vi "hardware_close_hardware.vi"(8 "error in (no error)":errorcluster, 11 "newport_xps in":refnum<class "newport_xps.lvclass">) -> (0 "error out":errorcluster, 3 "newport_xps out":refnum<class "newport_xps.lvclass">)   [LabVIEW 2015, in "newport_xps.lvclass"]
uses:
  newport_xps.lvclass
  newport_xps.lvclass/newport_xps.ctl
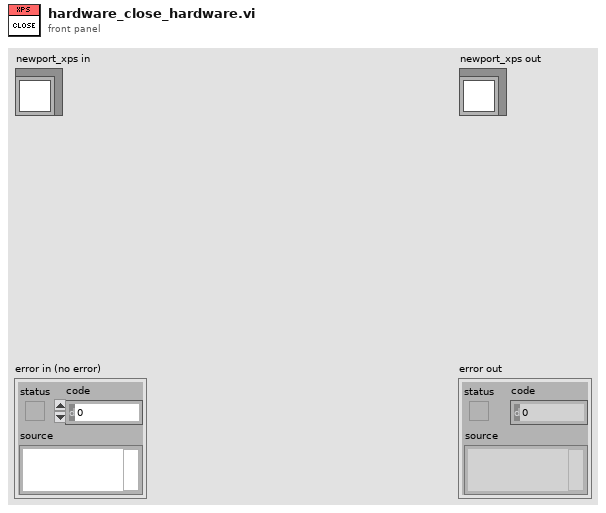
[diagram p1: front panel]
types:
  T1 = cluster{"connection TCP":refnum<k5>, "LogTo File":bool, "Log File refnum":refnum<file>, "no error if error log":bool}
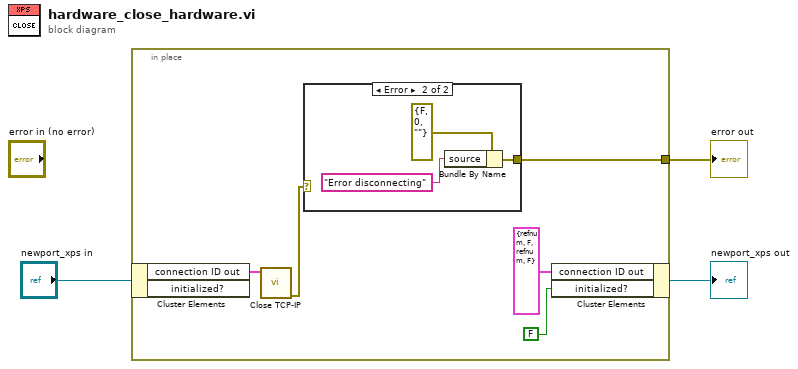
[diagram p0: block diagram]
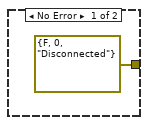
[diagram p2: hidden frame]
diagram:
  n1 = in-place {
    in-place-border: [w4] -> w2
    n2 = in-place-cluster #1("newport_xps in") -> ("connection ID out"=w8:T1)  [unwired: 1 out]
    n3 = call "Close TCP-IP.vi"("connection ID in"=w8) -> ("Error out"=w5:errorcluster)  [unwired: 10 in]
    n4 = case shown="Error" w5 {
      tunnel: [errorcluster {"status"=FALSE, "code"=0, "source"="Disconnected"} ("error IO") w11] -> w4
      frame No Error {
      }
      frame Error {
        n5 = Bundle By Name(cluster=errorcluster {"status"=FALSE, "code"=0, "source"=""} ("error IO"), "source"="Error disconnecting") -> (w11:errorcluster)
      }
    }
    n6 = in-place-cluster #1("connection ID out"=T1 {"connection TCP"=refnum, "LogTo File"=FALSE, "Log File refnum"=refnum, "no error if error log"=FALSE}, "initialized?"=FALSE) -> (→"newport_xps out":refnum<class "newport_xps.lvclass">)
  }
  "error out" <- w2
